vi "Create DAQmx Tasks.vi"(8 "Error In":errorcluster, 11 "Daqmx Module configuration":refnum<class "Daqmx Module configuration.lvclass">) -> (0 "Error Out":errorcluster, 2 "DAQ Tasks":T1)   [LabVIEW 2015, in "DAQmx Module Runtime.lvclass"]
doc: "Create unique tasks to be used in DCAF DAQmx module. Task names are based on module's UID and task type."
uses:
  DAQmx Module Runtime.lvclass
  DAQ Tasks.ctl
  configuration/Daqmx Module configuration.lvclass
  <vilib>/NI/Configuration Framework/serializable configuration/NISE_CEF_serializable configuration.lvclass/NISE_CEF_serializable configuration.ctl
  <vilib>/Utility/LVClass/Get LV Class Name.vi
  <vilib>/NI/Configuration Framework/error generator/NISE_error generator.vi
  <vilib>/NI/Configuration Framework/serializable configuration/NISE_CEF_serializable configuration.lvclass
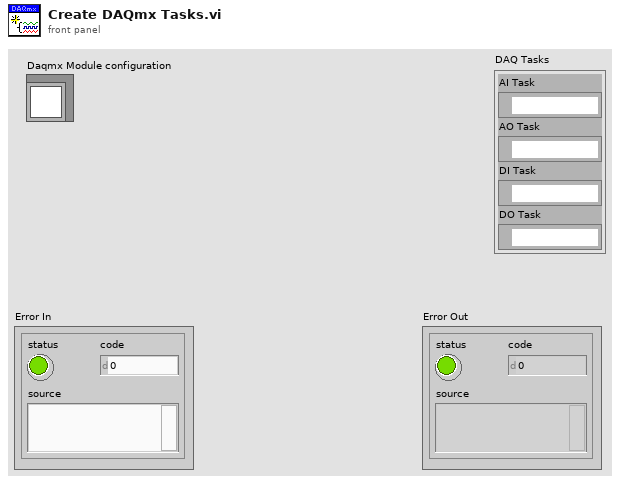
[diagram p1: front panel]
types:
  T1 = typedef "DAQmx Module Runtime.lvclass/DAQ Tasks.ctl" = cluster{"AI Task":refnum<k21>, "AO Task":refnum<k21>, "DI Task":refnum<k21>, "DO Task":refnum<k21>}
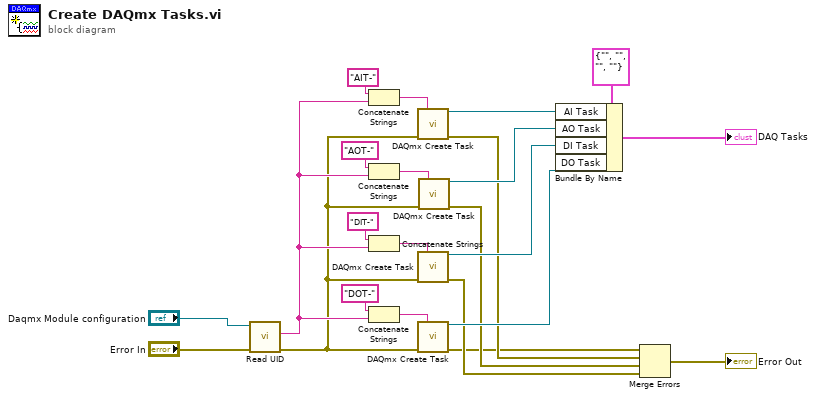
[diagram p0: block diagram]
diagram:
  n1 = call <vilib>:"Read UID.vi"("error in"="Error In", "configuration in"="Daqmx Module configuration") -> ("error out"=w1:errorcluster, "instance id"=w2:string)  [unwired: 7 in, 1 out]
  n2 = Concatenate Strings("AIT-" ("new task name"), w2) -> (w9:string)
  n3 = Concatenate Strings("AOT-" ("new task name"), w2) -> (w5:string)
  n4 = Concatenate Strings("DIT-" ("new task name"), w2) -> (w4:string)
  n5 = Concatenate Strings("DOT-" ("new task name"), w2) -> (w3:string)
  n6 = call <vilib>:"DAQmx Create Task.vi"("new task name"=w9, "error in"=w1) -> ("task out"=w22:refnum<k21>, "error out"=w16:errorcluster)  [unwired: 12 in]
  n7 = call <vilib>:"DAQmx Create Task.vi"("new task name"=w4, "error in"=w1) -> ("task out"=w20:refnum<k21>, "error out"=w18:errorcluster)  [unwired: 12 in]
  n8 = call <vilib>:"DAQmx Create Task.vi"("new task name"=w3, "error in"=w1) -> ("task out"=w19:refnum<k21>, "error out"=w15:errorcluster)  [unwired: 12 in]
  n9 = call <vilib>:"DAQmx Create Task.vi"("new task name"=w5, "error in"=w1) -> ("task out"=w21:refnum<k21>, "error out"=w17:errorcluster)  [unwired: 12 in]
  n10 = Bundle By Name(cluster=T1 {"AI Task"="", "AO Task"="", "DI Task"="", "DO Task"=""} ("DAQ Tasks"), "AI Task"=w22, "AO Task"=w21, "DI Task"=w20, "DO Task"=w19) -> (→"DAQ Tasks":T1)
  n11 = Merge Errors(w15, w16, w17, w18) -> (→"Error Out":errorcluster)
